vi "LENS_FEATURE_SELECTOR - Type.vi"(8 "error in (no error)":errorcluster) -> (0 "error out":errorcluster, 3 "LENS_FEATURE_SELECTOR_VALUE":i32)   [LabVIEW 2013]
doc: "<b>Buffer policy settings can be only unsafe in xiAPI LabVIEW library</b>\nUNSAFE : User gets pointer to internally allocated circle buffer and data may be overwritten by device.\nSAFE : Data from device will be copied to user allocated buffer or xiApi allocated memory."
uses:
  LENS_FEATURE_SELECTOR.ctl
  C:/Projects/Cameras3.x/xiLib/xiLIB_64bit/xiLIB/xiCamLib/API/x64/xiApi.NETX64.dll
  xiLIB_64bit/xiLIB/xiCamLib/API/x64/xiApi.NETX64.dll
panel:
  in  "LENS_FEATURE_SELECTOR":T1
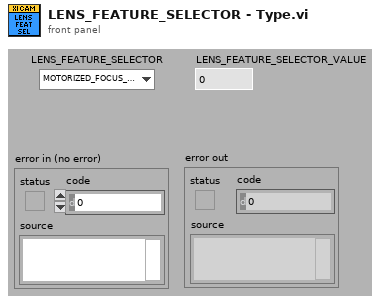
[diagram p1: front panel]
types:
  T1 = typedef "LENS_FEATURE_SELECTOR.ctl" = enum16{"MOTORIZED_FOCUS_SWITCH", "MOTORIZED_FOCUS_BOUNDED", "MOTORIZED_FOCUS_CALIBRATION", "IMAGE_STABILIZATION_ENABLED", "IMAGE_STABILIZATION_SWITCH_STATUS", "IMAGE_ZOOM_SUPPORTED"}
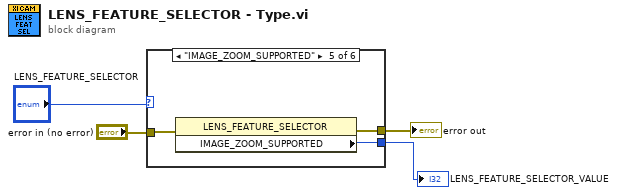
[diagram p0: block diagram]
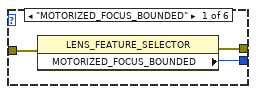
[diagram p2: hidden frame]
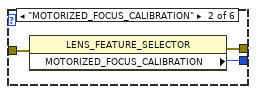
[diagram p3: hidden frame]
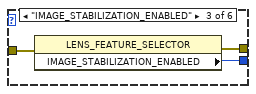
[diagram p4: hidden frame]
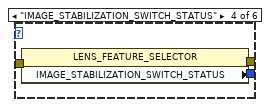
[diagram p5: hidden frame]
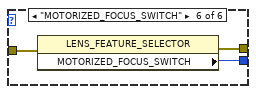
[diagram p6: hidden frame]
diagram:
  n1 = case shown="\"IMAGE_ZOOM_SUPPORTED\"" "LENS_FEATURE_SELECTOR" {
    tunnel: "error in (no error)" -> [w7 w10 w13 w16 w19 w22]
    tunnel: [w6 w9 w12 w15 w18 w21] -> w3
    tunnel: [w5 w8 w11 w14 w17 w20] -> w2
    frame "MOTORIZED_FOCUS_BOUNDED" {
      n2 = property class="LENS_FEATURE_SELECTOR"(error in=w7) -> (error out=w6:errorcluster, "MOTORIZED_FOCUS_BOUNDED"=w5:i32)  [unwired: 1 in, 1 out]
    }
    frame "MOTORIZED_FOCUS_CALIBRATION" {
      n3 = property class="LENS_FEATURE_SELECTOR"(error in=w10) -> (error out=w9:errorcluster, "MOTORIZED_FOCUS_CALIBRATION"=w8:i32)  [unwired: 1 in, 1 out]
    }
    frame "IMAGE_STABILIZATION_ENABLED" {
      n4 = property class="LENS_FEATURE_SELECTOR"(error in=w13) -> (error out=w12:errorcluster, "IMAGE_STABILIZATION_ENABLED"=w11:i32)  [unwired: 1 in, 1 out]
    }
    frame "IMAGE_STABILIZATION_SWITCH_STATUS" {
      n5 = property class="LENS_FEATURE_SELECTOR"(error in=w16) -> (error out=w15:errorcluster, "IMAGE_STABILIZATION_SWITCH_STATUS"=w14:i32)  [unwired: 1 in, 1 out]
    }
    frame "IMAGE_ZOOM_SUPPORTED" {
      n6 = property class="LENS_FEATURE_SELECTOR"(error in=w19) -> (error out=w18:errorcluster, "IMAGE_ZOOM_SUPPORTED"=w17:i32)  [unwired: 1 in, 1 out]
    }
    frame "MOTORIZED_FOCUS_SWITCH" {
      n7 = property class="LENS_FEATURE_SELECTOR"(error in=w22) -> (error out=w21:errorcluster, "MOTORIZED_FOCUS_SWITCH"=w20:i32)  [unwired: 1 in, 1 out]
    }
  }
  "error out" <- w3
  "LENS_FEATURE_SELECTOR_VALUE" <- w2
